vi "그림 6-3-5 아스키 파일 읽기.vi"() -> ()   [LabVIEW 2010]
panel:
  out "텍스트":string
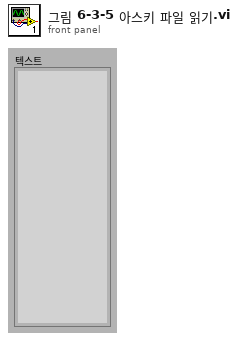
[diagram p1: front panel]
types:
  T1 = enum16{"open", "replace", "create", "open or create", "replace or create", "replace or create with confirmation"}
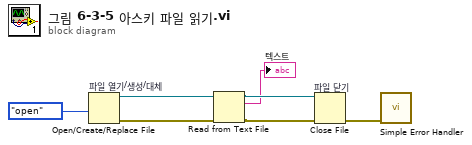
[diagram p0: block diagram]
diagram:
  n1 = Open/Create/Replace File "파일 열기/생성/대체"(operation (0:open)=T1."open" ("동작(0:open)")) -> (refnum out=w5:refnum<file>, error out=w4:errorcluster)  [unwired: 5 in, 1 out]
  n2 = Read from Text File(file (use dialog)=w5, error in=w4) -> (refnum out=w3:refnum<file>, text=→"텍스트":string, error out=w2:errorcluster)  [unwired: 2 in, 1 out]
  n3 = Close File "파일 닫기"(refnum=w3, error in=w2) -> (error out=w7:errorcluster)  [unwired: 1 out]
  n4 = call <vilib>:"Simple Error Handler.vi"("error in (no error)"=w7) -> ()  [unwired: 4 in, 5 out]
